vi "Get Targets.vi"(8 "error in (no error)":errorcluster, 10 "Targeting Units":T2(array[cluster]), 11 "Target in [pix]":T1(array[cluster])) -> (0 "error out":errorcluster, 2 "Objects to track Out [pix]":cluster{"X":dbl, "Y":dbl}[](array[cluster]))   [LabVIEW 2012, in "Visual Analyser.lvlib"]
uses:
  Visual Analyser.lvlib
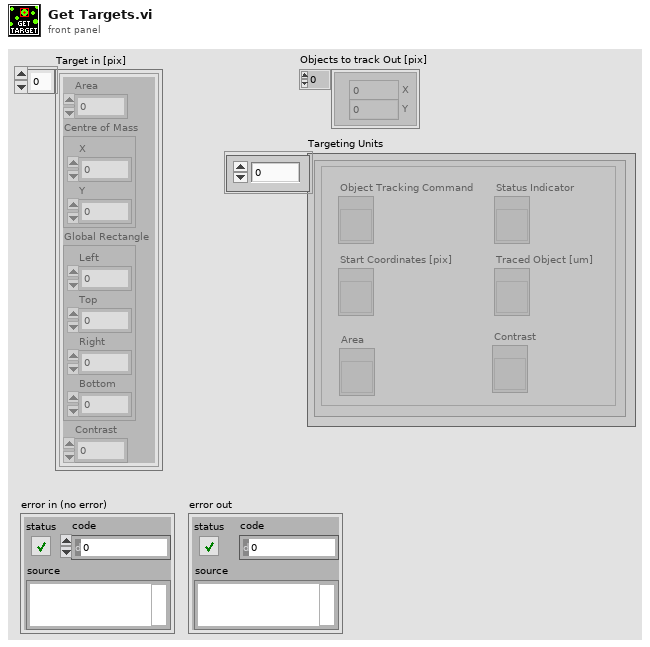
[diagram p1: front panel]
types:
  T1 = cluster{"Area":dbl, "Centre of Mass":cluster{"X":dbl, "Y":dbl}, "Global Rectangle":cluster{"Left":dbl, "Top":dbl, "Right":dbl, "Bottom":dbl}, "Contrast":dbl}[]
  T2 = cluster{"Object Tracking Command":refnum<vi>, "Status Indicator":refnum<vi>, "Start Coordinates [pix]":refnum<vi>, "Traced Object [um]":refnum<vi>, "Area":refnum<vi>, "Contrast":refnum<vi>}[]
  T3 = cluster{"Area":dbl, "Centre of Mass":cluster{"X":dbl, "Y":dbl}, "Global Rectangle":cluster{"Left":dbl, "Top":dbl, "Right":dbl, "Bottom":dbl}, "Contrast":dbl}
  T4 = cluster{"Left":dbl, "Top":dbl, "Right":dbl, "Bottom":dbl}
  T5 = cluster{"Left":bool, "Top":bool, "Right":bool, "Bottom":bool}
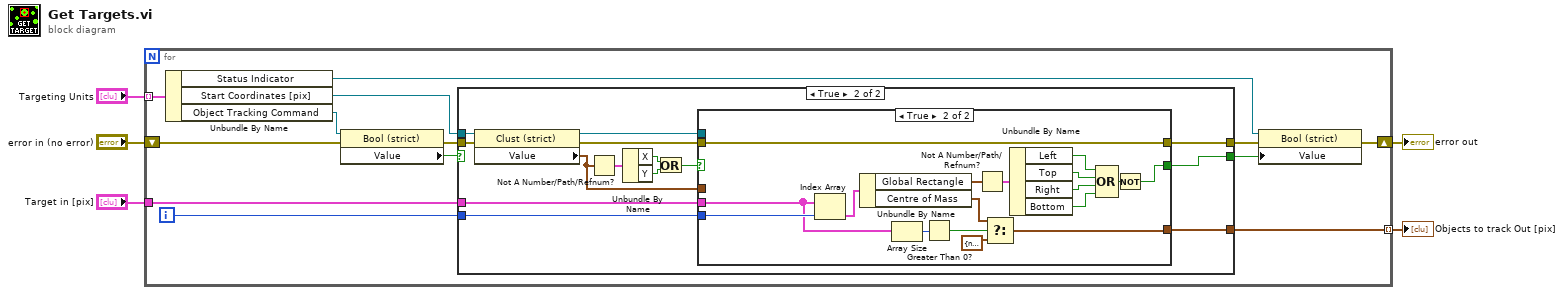
[diagram p0: block diagram]
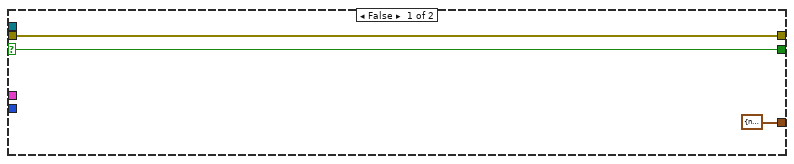
[diagram p2: hidden frame]
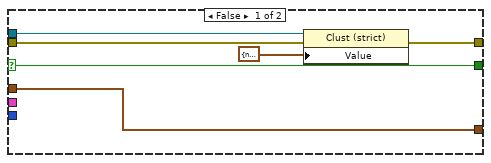
[diagram p3: hidden frame]
diagram:
  n1 = for {
    tunnel: "Targeting Units" -> [w18] mode=indexing
    shift-right: [w8] -> w5
    shift-left: "error in (no error)" -> [w15]
    tunnel: "Target in [pix]" -> [w6]
    tunnel: [w11] -> w3 mode=indexing
    i -> [w7]
    n2 = Unbundle By Name(w18) -> ("Status Indicator"=w10:refnum<vi>, "Start Coordinates [pix]"=w17:refnum<vi>, "Object Tracking Command"=w13:refnum<vi>)
    n3 = property class="Bool (strict)"(reference=w13, error in=w15) -> (error out=w14:errorcluster, "Value"=w12:bool)  [unwired: 1 out]
    n4 = case shown="True" w12 {
      selector: w12 -> [w21 _]
      tunnel: w17 -> [_ w35]
      tunnel: w14 -> [w20 w27]
      tunnel: [w21 w26] -> w16
      tunnel: [w20 w24] -> w9
      tunnel: w6 -> [_ w25]
      tunnel: [cluster{"X":dbl, "Y":dbl} {"X"=nan, "Y"=nan} ("Centre of Mass") w23] -> w11
      tunnel: w7 -> [_ w22]
      frame False {
      }
      frame True {
        n5 = property class="Clust (strict)"(reference=w35, error in=w27) -> (reference out=w31:refnum<vi>, error out=w30:errorcluster, "Value"=w28:cluster{"X":dbl, "Y":dbl})
        n6 = Not A Number/Path/Refnum?(number/path/refnum=w28) -> (NaN/Path/Refnum?=w34:cluster{"X":bool, "Y":bool})
        n7 = Unbundle By Name(w34) -> ("X"=w32:bool, "Y"=w33:bool)
        n8 = Or(x=w32, y=w33) -> (x .or. y?=w29:bool)
        n9 = case shown="True" w29 {
          selector: w29 -> [w38 _]
          tunnel: w31 -> [w41 _]
          tunnel: w30 -> [w40 w58]
          tunnel: [w36 w44] -> w23
          tunnel: w28 -> [w36 _]
          tunnel: [w39 w58] -> w24
          tunnel: w25 -> [_ w46]
          tunnel: [w38 w50] -> w26
          tunnel: w22 -> [_ w49]
          frame False {
            n10 = property class="Clust (strict)"(reference=w41, error in=w40, "Value"=cluster{"X":dbl, "Y":dbl} {"X"=nan, "Y"=nan} ("Point Coordinates")) -> (error out=w39:errorcluster)  [unwired: 1 out]
          }
          frame True {
            n11 = Index Array(array=w46, index=w49) -> (element=w48:T3)
            n12 = Unbundle By Name(w48) -> ("Global Rectangle"=w51:T4, "Centre of Mass"=w43:cluster{"X":dbl, "Y":dbl})
            n13 = Array Size(array=w46) -> (size(s)=w47:i32)
            n14 = Greater Than 0?(x=w47) -> (x > 0?=w45:bool)
            n15 = Not A Number/Path/Refnum?(number/path/refnum=w51) -> (NaN/Path/Refnum?=w53:T5)
            n16 = Select(t=w43, s=w45, f=cluster{"X":dbl, "Y":dbl} {"X"=nan, "Y"=nan} ("Point Coordinates")) -> (s? t:f=w44:cluster{"X":dbl, "Y":dbl})
            n17 = Unbundle By Name(w53) -> ("Left"=w54:bool, "Top"=w55:bool, "Right"=w56:bool, "Bottom"=w57:bool)
            n18 = Compound Arithmetic op=OR(w54, w55, w56, w57) -> (w52:bool)
            n19 = Not(x=w52) -> (.not. x?=w50:bool)
          }
        }
      }
    }
    n20 = property class="Bool (strict)"(reference=w10, error in=w9, "Value"=w16) -> (error out=w8:errorcluster)  [unwired: 1 out]
  }
  "error out" <- w5
  "Objects to track Out [pix]" <- w3
